vi "Find Workspace.vi"(8 "error in (no error)":errorcluster, 9 "Type of Hexaboard":T1, 10 "Control In":T3={"I-O.lvclass"=refnum, "Gantry"=refnum, "Dispenser"="COM1"}, 11 "Component.lvclass":refnum<class "Component Tray.lvclass">) -> (0 "error out":errorcluster, 1 "Workspace":T2, 2 "Control Out":T3={"I-O.lvclass"=refnum, "Gantry"=refnum, "Dispenser"="COM1"}, 3 "Workspace Out":refnum<class "Component Tray.lvclass">)   [LabVIEW 2021, in "Component Tray.lvclass"]
uses:
  Component Tray.lvclass
  Controller/Controllers.ctl
  Controller/I-O/I-O.lvclass
  C:/Program Files (x86)/Aerotech/A3200/LabVIEW/2010/Bin/Aerotech.A3200.dll
  Program Files (x86)/Aerotech/A3200/LabVIEW/2010/Bin/Aerotech.A3200.dll
  Workspace.ctl
  C:/Users/hep/Documents/UCSB-CMU-GantryCode/UCSB-Gantry-HEP-main (3)/UCSB-Gantry-HEP-main/Classes/Workspace/Fixture.lvclass
  Routine/TypeOfHexaboard.ctl
  Fixture.lvclass/Fixture.ctl
  Read Fixture ID.vi
  Read Position.vi
  Fixture.lvclass
  Controller/Controller.lvclass
  Routine/Routine.lvclass
panel:
  out "XYZTheta":dbl[](array[numeric]) format="%#.6g"
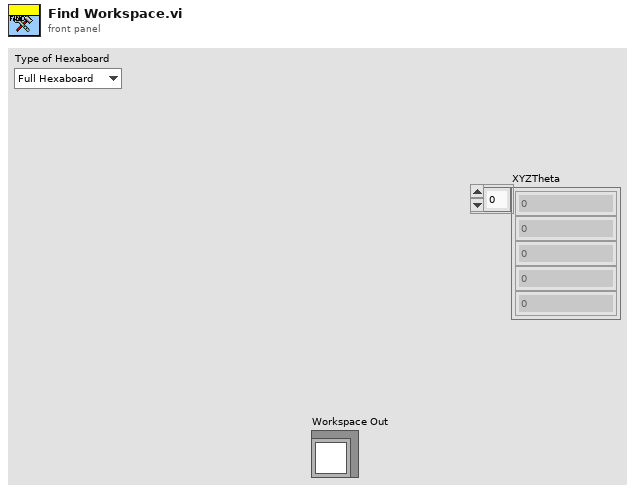
[diagram p1: front panel]
types:
  T1 = typedef "Routine.lvclass/TypeOfHexaboard.ctl" = enum16{"Full Hexaboard", "Right Partial PCB", "Right Partial Sensor", "Al Dummy Right Partial Sensor"}
  T2 = typedef "Fixture.lvclass/Workspace.ctl" = cluster{"XYZTheta":dbl[], "Workspace Valve":i32, "Workspace Sensor":i32}
  T3 = typedef "Controller.lvclass/Controllers.ctl" = cluster{"I-O.lvclass":refnum<class "I-O.lvclass">, "Gantry":refnum<k24>, "Dispenser":refnum<visa-resource-name>}
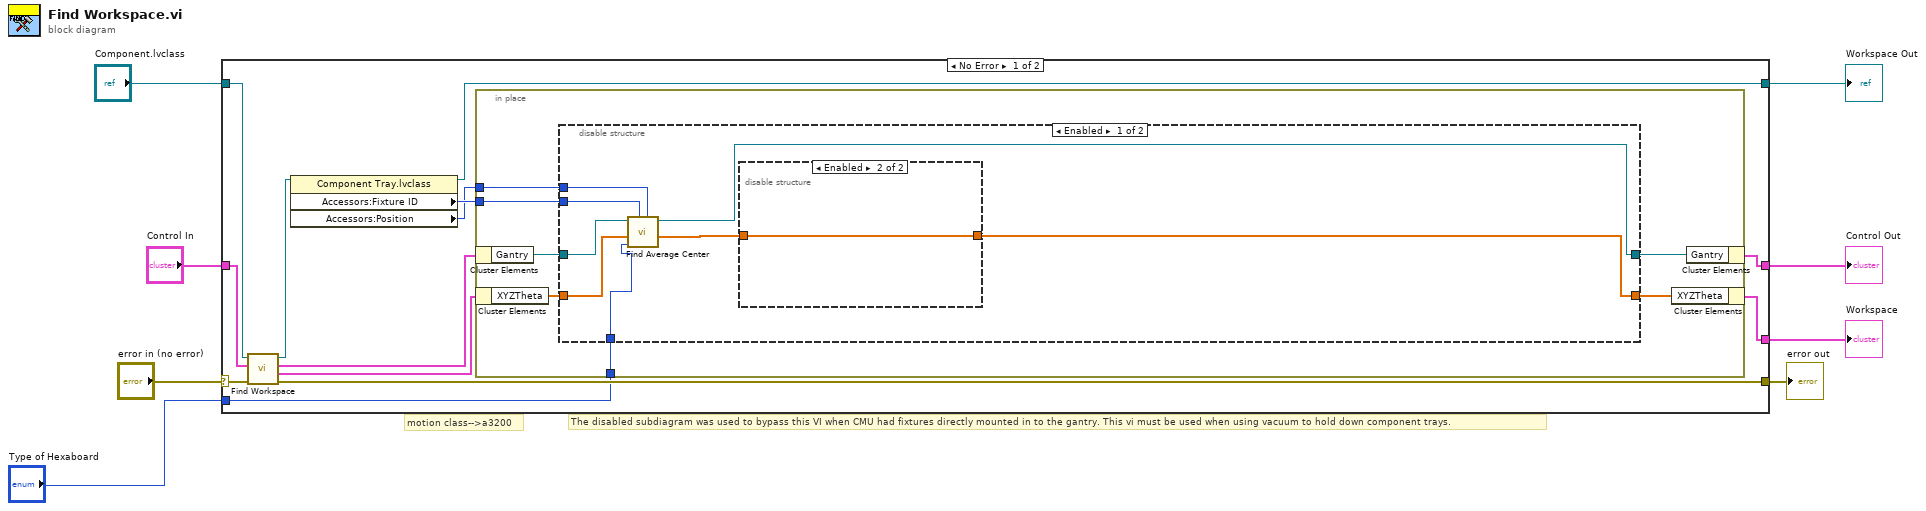
[diagram p0: block diagram]
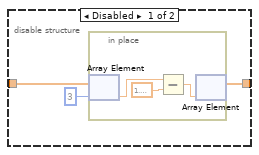
[diagram p2: hidden frame]
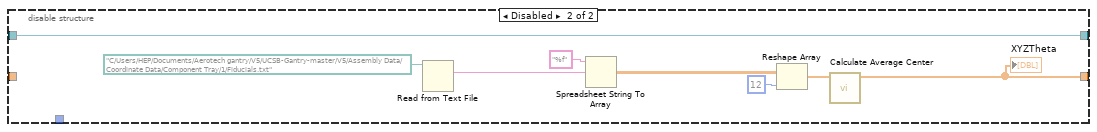
[diagram p3: hidden frame]
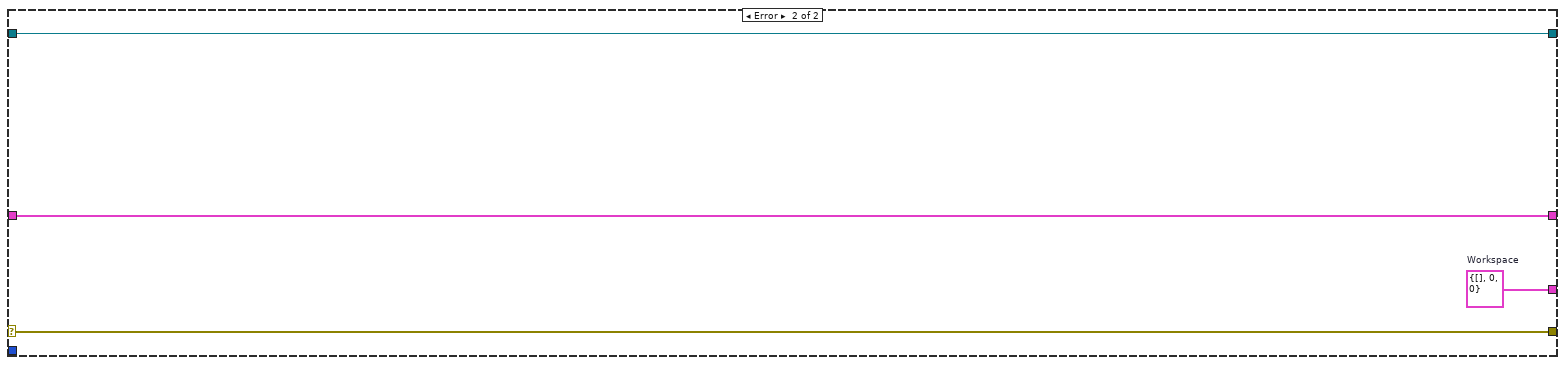
[diagram p4: hidden frame]
diagram:
  # "The disabled subdiagram was used to bypass this VI when CMU had fixtures directly mounted in to the gantry. This vi must be used when using vacuum to hold down component trays."
  # "motion class-->a3200"
  n1 = case shown="No Error" "error in (no error)" {
    selector: "error in (no error)" -> [w19 w55]
    tunnel: [w15 w54] -> w8
    tunnel: [w21 w55] -> w7
    tunnel: [w14 w53] -> w6
    tunnel: "Control In" -> [w18 w54]
    tunnel: [w11 w52] -> w3
    tunnel: "Component.lvclass" -> [w17 w52]
    tunnel: "Type of Hexaboard" -> [w10 _]
    frame No Error {
      n2 = call-parent "Find Workspace.vi"("Error In"=w19, "Control In"=w18, "Workspace In"=w17) -> ("Error Out"=w21:errorcluster, 1:"Workspace Out"=w20:T2, "Control Out"=w16:T3, 3:"Workspace Out"=w12:refnum<class "Component Tray.lvclass">)  [unwired: 5 in]
      n3 = property class="Component Tray.lvclass"(reference=w12) -> (reference out=w11:refnum<class "Component Tray.lvclass">, "Accessors:Fixture ID"=w13:i32, "Accessors:Position"=w9:i32)  [unwired: 1 in, 1 out]
      n4 = in-place {
        in-place-border: w13 -> [w27]
        in-place-border: w9 -> [w28]
        in-place-border: w10 -> [w22]
        n5 = in-place-cluster #1(w16) -> ("Gantry"=w26:refnum<k24>)
        n6 = in-place-cluster #2(w20) -> ("XYZTheta"=w25:dbl[])
        n7 = disable-structure shown="Enabled" {
          disable-tunnel: w28 -> [w33 _]
          disable-tunnel: w27 -> [w32 _]
          disable-tunnel: w26 -> [w36 w44]
          disable-tunnel: w25 -> [w35 _]
          disable-tunnel: [w30 w45] -> w24
          disable-tunnel: [w34 w44] -> w23
          disable-tunnel: w22 -> [w29 _]
          frame Enabled {
            n8 = call "Find Average Center.vi"("Position"=w33, "Tray Number"=w32, "Type of Hexaboard"=w29, "XYZTheta"=w35, "Gantry In"=w36) -> ("XYZTheta"=w31:dbl[], "Gantry Out"=w34:refnum<k24>)  [unwired: 5 in]
            n9 = disable-structure shown="Enabled" {
              disable-tunnel: w31 -> [w39 w43]
              disable-tunnel: [w37 w43] -> w30
              frame Disabled {
                n10 = in-place {
                  n11 = in-place-array #3(w39, 3) -> (w42:dbl)
                  n12 = Subtract(x=w42, y=1.5707963267948966) -> (x-y=w40:dbl)
                  n13 = in-place-array #3(w40) -> (w37:dbl[])  [unwired: 1 out]
                }
              }
              frame Enabled {
              }
            }
          }
          frame Disabled {
            n14 = Read from Text File(file (use dialog)=path "C:/Users/HEP/Documents/Aerotech gantry/V5/UCSB-Gantry-master/V5/Assembly Data/Coordinate Data/Component Tray/1/Fiducials.txt") -> (text=w49:string)  [unwired: 3 in, 3 out]
            n15 = Spreadsheet String To Array(format string="%f", spreadsheet string=w49) -> (array=w48:dbl[][])  [unwired: 2 in]
            n16 = Reshape Array(w48, 12 ("dimension size")) -> (w46:dbl[])
            n17 = call "Calculate Average Center.vi"("Gantry Fiducials"=w46) -> ("XYZTheta"=w45:dbl[])  [unwired: 8 in, 2 out]
            "XYZTheta" <- w45
          }
        }
        n18 = in-place-cluster #2("XYZTheta"=w24) -> (w14:T2)
        n19 = in-place-cluster #1("Gantry"=w23) -> (w15:T3)
      }
    }
    frame Error {
      w53 = T2 {"XYZTheta"=[], "Workspace Valve"=0, "Workspace Sensor"=0}  # Workspace
    }
  }
  "error out" <- w7
  "Control Out" <- w8
  "Workspace" <- w6
  "Workspace Out" <- w3
